vi "TankDrive.vi"(8 "error in":errorcluster, 10 "Right Value":dbl, 11 "Left Value":dbl) -> (0 "error out":errorcluster)   [LabVIEW 2016]
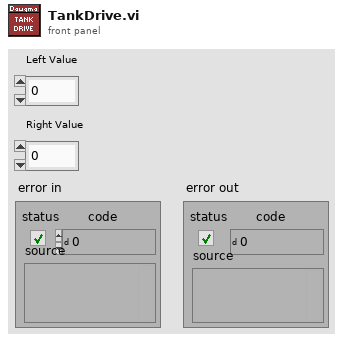
[diagram p1: front panel]
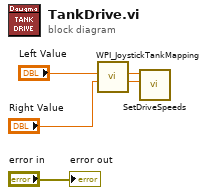
[diagram p0: block diagram]
diagram:
  n1 = call <vilib>:"WPI_JoystickTankMapping.vi"("Right axis value"="Right Value", "Left axis value"="Left Value") -> ("Right Motor Value"=w1:dbl, "Left Motor Value"=w2:dbl)  [unwired: 8 in]
  n2 = call "SetDriveSpeeds.vi"("Right Value"=w1, "Left Value"=w2) -> ()  [unwired: 9 in, 1 out]
  "error out" <- "error in"
